vi "Read Message.vi"(6 "timeout ms (25000)":i32, 8 "error in (no error)":errorcluster, 11 "GenNet Variant Protocol in":refnum<class "GenNet Variant Protocol.lvclass">) -> (0 "error out":errorcluster, 2 "Message":variant, 3 "GenNet Variant Protocol out":refnum<class "GenNet Variant Protocol.lvclass">)   [LabVIEW 2020, in "hse-gennet.lvlib" / "GenNet Variant Protocol.lvclass"]
doc: "____\nHAMPEL SOFTWARE ENGINEERING v3.8.0 (2023-12-18 14:41)"
uses:
  GenNet Variant Protocol.lvclass
  C:/GitLab-Runner/builds/7NHnU7RQc/0/open-source/hse-libraries/Source/hse-gennet/GenNet Protocols/GenNet Protocol.lvclass
  GenNet Protocol.lvclass/GenNet Protocol.ctl
  Get Connection ID.vi
  GenNet Variant Protocol.lvclass/GenNet Variant Protocol.ctl
  hse-gennet.lvlib
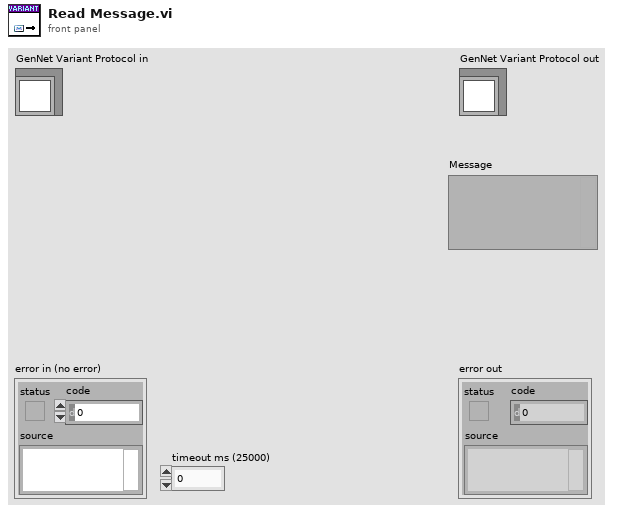
[diagram p1: front panel]
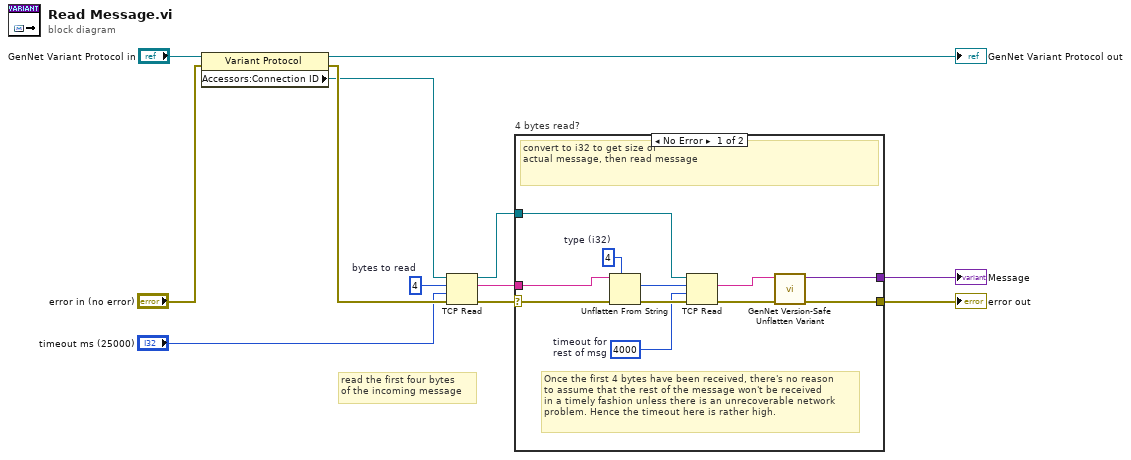
[diagram p0: block diagram]
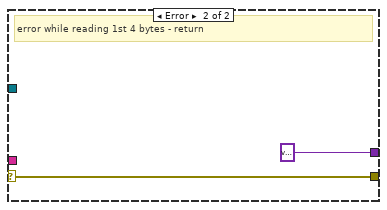
[diagram p2: hidden frame]
diagram:
  w10 = 4  # bytes to read
  # "read the first four bytes\nof the incoming message"
  n1 = property class="Variant Protocol"(reference="GenNet Variant Protocol in", error in="error in (no error)") -> (reference out=→"GenNet Variant Protocol out":refnum<class "GenNet Variant Protocol.lvclass">, error out=w5:errorcluster, "Accessors:Connection ID"=w4:refnum<k5>)
  n2 = TCP Read(connection ID=w4, bytes to read=w10, error in (no error)=w5, 9:"timeout ms (25000)") -> (connection ID out=w8:refnum<k5>, data out=w9:string, error out=w7:errorcluster)  [unwired: 1 in]
  n3 = case "4 bytes read?" shown="No Error" w7 {
    selector: w7 -> [w17 w25]
    tunnel: w9 -> [w23 _]
    tunnel: w8 -> [w19 _]
    tunnel: [w15 w25] -> w6
    tunnel: [w14 variant] -> w2
    frame No Error {
      w22 = 4  # type (i32)
      w18 = 4000  # timeout for  rest of msg
      # "Once the first 4 bytes have been received, there's no reason\nto assume that the rest of the message won't be received\nin a timely fashion unless there is an unrecoverable network\nproblem. Hence the timeout here is rather high."
      # "convert to i32 to get size of\nactual message, then read message"
      n4 = Unflatten From String(type=w22, binary string=w23, error in (no error)=w17) -> (value=w21:i32, error out=w20:errorcluster)  [unwired: 2 in, 1 out]
      n5 = TCP Read(connection ID=w19, bytes to read=w21, error in (no error)=w20, 9:w18) -> (data out=w13:string, error out=w16:errorcluster)  [unwired: 1 in, 1 out]
      n6 = call "GenNet Version-Safe Unflatten Variant.vi"("error in"=w16, "Flattened Data"=w13) -> ("error out"=w15:errorcluster, "Message Data"=w14:variant)  [unwired: 8 in]
    }
    frame Error {
      # "error while reading 1st 4 bytes - return"
    }
  }
  "error out" <- w6
  "Message" <- w2
